vi "EnQueue Actions with Data.vi"(0 "action queue in":refnum<queue>, 5 "action and data":T1[](array[typedef]), 11 "error in":errorcluster) -> (4 "action queue out":refnum<queue>, 15 "error out":errorcluster)   [LabVIEW 2026, in "Synchronize AWS S3 Content.lvlib" / "Actions.lvlib"]
doc: "Adds multiple elements to the action queue.\n\n<B>Input Parameters</B>\n\n<B>action queue in</B> is a reference to a queue. Use the Create Action Queue function to obtain a queue reference. \n\n<B>action and data</B> inserted into system.\n\n<B>error in</B> describes error conditions that occur before this node runs. This input provides standard error in functionality.\n\n<B>Output Parameters</B>\n\n<B>action queue out</B> returns the reference to the queue unchanged. \n\n<B>error out</B> contains error information. This output provides standard error out functionality."
uses:
  Actions.lvlib
  System Action Element.ctl
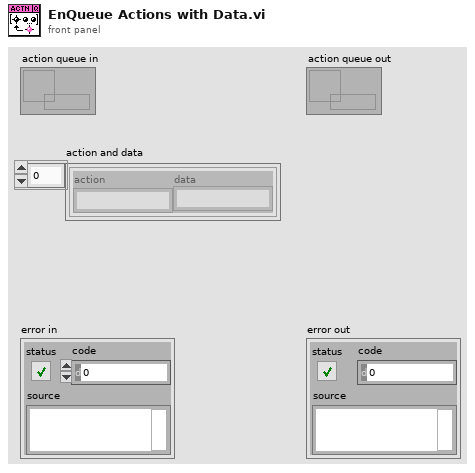
[diagram p1: front panel]
types:
  T1 = typedef "Synchronize AWS S3 Content.lvlib/Actions.lvlib/System Action Element.ctl" = cluster{"action":string, "data":string}
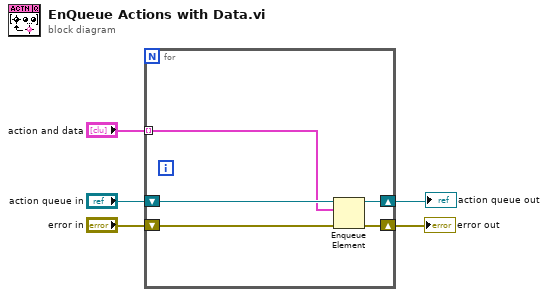
[diagram p0: block diagram]
diagram:
  n1 = for {
    shift-right: [w9] -> w4
    shift-left: "error in" -> [w10]
    shift-right: [w7] -> w2
    shift-left: "action queue in" -> [w8]
    tunnel: "action and data" -> [w6] mode=indexing
    n2 = Enqueue Element(queue=w8, element=w6, error in (no error)=w10) -> (queue out=w7:refnum<queue>, error out=w9:errorcluster)  [unwired: 1 in, 1 out]
  }
  "error out" <- w4
  "action queue out" <- w2
